vi "Test DI and DO with Troubleshooter.vi"() -> ()   [LabVIEW 2013]
uses:
  SLL DAQ Engine/Software/Source Code/Sub VIs/DAQ Engine/Controls/SLL DE DI Global Options.ctl
  SLL DAQ Engine/Software/Source Code/Sub VIs/DAQ Engine/Controls/SLL DE DO Global Options.ctl
  Controls/ALTS-2015 LV2GBL Station Info Options.ctl
  SLL DAQ Engine/Software/Source Code/Sub VIs/DAQ Engine/Controls/SLL DE List of Digital Inputs.ctl
  SLL DAQ Engine/Software/Source Code/Sub VIs/DAQ Engine/Controls/SLL DE List of Digital Outputs.ctl
  Controls/ALTS-2015 Auto Program States.ctl
panel:
  out "St4 Select Test":bool
  out "St3 Select Test":bool
  out "St2 Select Test":bool
  out "St1 Select Test":bool
  out "St4 Status":bool caption="Status"
  out "St4 Start/Stop":bool
  in  "STATION4 TC FAIL":bool
  in  "STATION4 TC PASS":bool
  out "St4 Test Result":bool caption="Test Result"
  in  "STATION4 Test Type":T1(ring)
  in  "STATION4 Clamped":bool
  in  "STATION4 Stop":bool
  in  "STATION4 Start":bool
  out "St2 Status":bool caption="Status"
  out "St2 Start/Stop":bool
  in  "STATION2 TC FAIL":bool
  in  "STATION2 TC PASS":bool
  out "St2 Test Result":bool caption="Test Result"
  in  "STATION2 Test Type":T1(ring)
  in  "STATION2 Clamped":bool
  in  "STATION2 Stop":bool
  in  "STATION2 Start":bool
  out "St3 Status":bool caption="Status"
  out "St3 Start/Stop":bool
  in  "STATION3 TC FAIL":bool
  in  "STATION3 TC PASS":bool
  out "St3 Test Result":bool caption="Test Result"
  in  "STATION3 Test Type":T1(ring)
  in  "STATION3 Clamped":bool
  in  "STATION3 Stop":bool
  in  "STATION3 Start":bool
  in  "Enum":T2=enum."Write Task Available for Robot"
  in  "Trigger Robot Controller State":bool
  out "St1 Status":bool caption="Status"
  in  "PC ACK Read Tags":dbl
  out "Invalid Serial Number":bool
  out "Rerun?":bool
  out "Station Number":string
  out "Test Result":bool
  out "Serial Flange Size":string
  out "Serial Displacement Size":dbl
  out "Serial Adapter Plate Size":dbl
  out "New Serial Task?":bool
  out "Task Available for Robot?":bool
  in  "Robot Available":bool
  in  "Station No Start Stop Test":T3(ring)
  in  "Scan Trigger":bool
  in  "Stop Test":bool
  in  "Start Test":bool
  out "St1 Start/Stop":bool
  in  "STATION1 TC FAIL":bool
  in  "STATION1 TC PASS":bool
  out "St1 Test Result":bool caption="Test Result"
  in  "STATION1 Test Type":T1(ring)
  in  "STATION1 Clamped":bool
  in  "STATION1 Stop":bool
  in  "STATION1 Start":bool
  out "Station Number":string
  in  "PC_ACK_Read_Tags":dbl
  out "Test Type":i32
  out "DO Channel Name":T4
  out "String":string
  in  "Invalid_SNo":dbl
  in  "Station_No_Start_Stop_Test":dbl
  in  "Start_Test":dbl
  in  "Rerun":dbl
  in  "Station_Number":dbl
  in  "Test_Result":dbl
  in  "Serial_Flange_Size":string
  in  "Serial_Displacement_Size":dbl
  in  "Serial_Adapter_Size":dbl
  in  "New_Serial":dbl
  in  "Scan_Trigger":dbl
  in  "Stop_Test":dbl
  in  "Task_Available_for_Robot":dbl
  in  "Robot_Available":dbl
  in  "DI Array":bool[](array[boolean])=[FALSE, FALSE, FALSE, FALSE, FALSE, FALSE, FALSE, FALSE, FALSE, FALSE, FALSE, FALSE, FALSE, FALSE, FALSE, FALSE, FALSE, FALSE, FALSE, FALSE, FALSE, FALSE, FALSE, FALSE, FALSE, FALSE, FALSE, FALSE]
  in  "DI Channel Name Array":T5[](array[typedef])=[enum."STATION1_START", enum."STATION1_STOP", enum."STATION1_CLAMPED", enum."STATION1_TC_PASS", enum."STATION1_TC_FAIL", enum."STATION1_TTA", enum."STATION1_TTB", enum."STATION2_START", enum."STATION2_STOP", enum."STATION2_CLAMPED", enum."STATION2_TC_PASS", enum."STATION2_TC_FAIL", enum."STATION2_TTA", enum."STATION2_TTB", enum."STATION3_START", enum."STATION3_STOP", enum."STATION3_CLAMPED", enum."STATION3_TC_PASS", enum."STATION3_TC_FAIL", enum."STATION3_TTA", enum."STATION3_TTB", enum."STATION4_START", enum."STATION4_STOP", enum."STATION4_CLAMPED", enum."STATION4_TC_PASS", enum."STATION4_TC_FAIL", enum."STATION4_TTA", enum."STATION4_TTB"]
  out "DO Channel Name Array":T4[](array[typedef])=[enum."STATION1_START TEST", enum."STATION1_STOP TEST", enum."STATION1_LIGHT1", enum."STATION1_LIGHT2", enum."STATION1_LIGHT3", enum."STATION1_SELECT_TEST", enum."STATION2_START TEST", enum."STATION2_STOP TEST", enum."STATION2_LIGHT1", enum."STATION2_LIGHT2", enum."STATION2_LIGHT3", enum."STATION2_SELECT_TEST", enum."STATION3_START TEST", enum."STATION3_STOP TEST", enum."STATION3_LIGHT1", enum."STATION3_LIGHT2", enum."STATION3_LIGHT3", enum."STATION3_SELECT_TEST", enum."STATION4_START TEST", enum."STATION4_STOP TEST", enum."STATION4_LIGHT1", enum."STATION4_LIGHT2", enum."STATION4_LIGHT3", enum."STATION4_SELECT_TEST"]
  out "DO Status":bool[](array[boolean])
  out "error out":errorcluster
  in  "error in":errorcluster
  in  "DI Channel Name":T5
  in  "stop":bool
  # "STATION  1"
  # "STATION  2"
  # "Write Tags\nPC Writes to PLC\nPLC can only read these tags"
  # "Read Tags\nPC Reads from PLC"
  # "DO"
  # "DO"
  # "DO"
  # "DO"
  # "STATION  3"
  # "STATION  4"
  # "DO"
  # "DO"
  # "DO"
  # "DO"
  # "TROUBLESHOOTER"
  # "Simulation VI to send DI Status and reads the DO output"
  # "Write Tags\nPC Writes to PLC\nPLC can only read these tags"
  # "Read Tags\nPC Reads from PLC"
  # "Test Type1: TTA:1, TTB: 0;\nTest Type2: TTA:0, TTB: 1;\nTest Type3: TTA:1, TTB: 1;\nTest Type4: TTA:0, TTB: 0;"
  # "IDLE : \t\t100\nTest Running:\t 010\nPass\t\t110\nFail\t\t101"
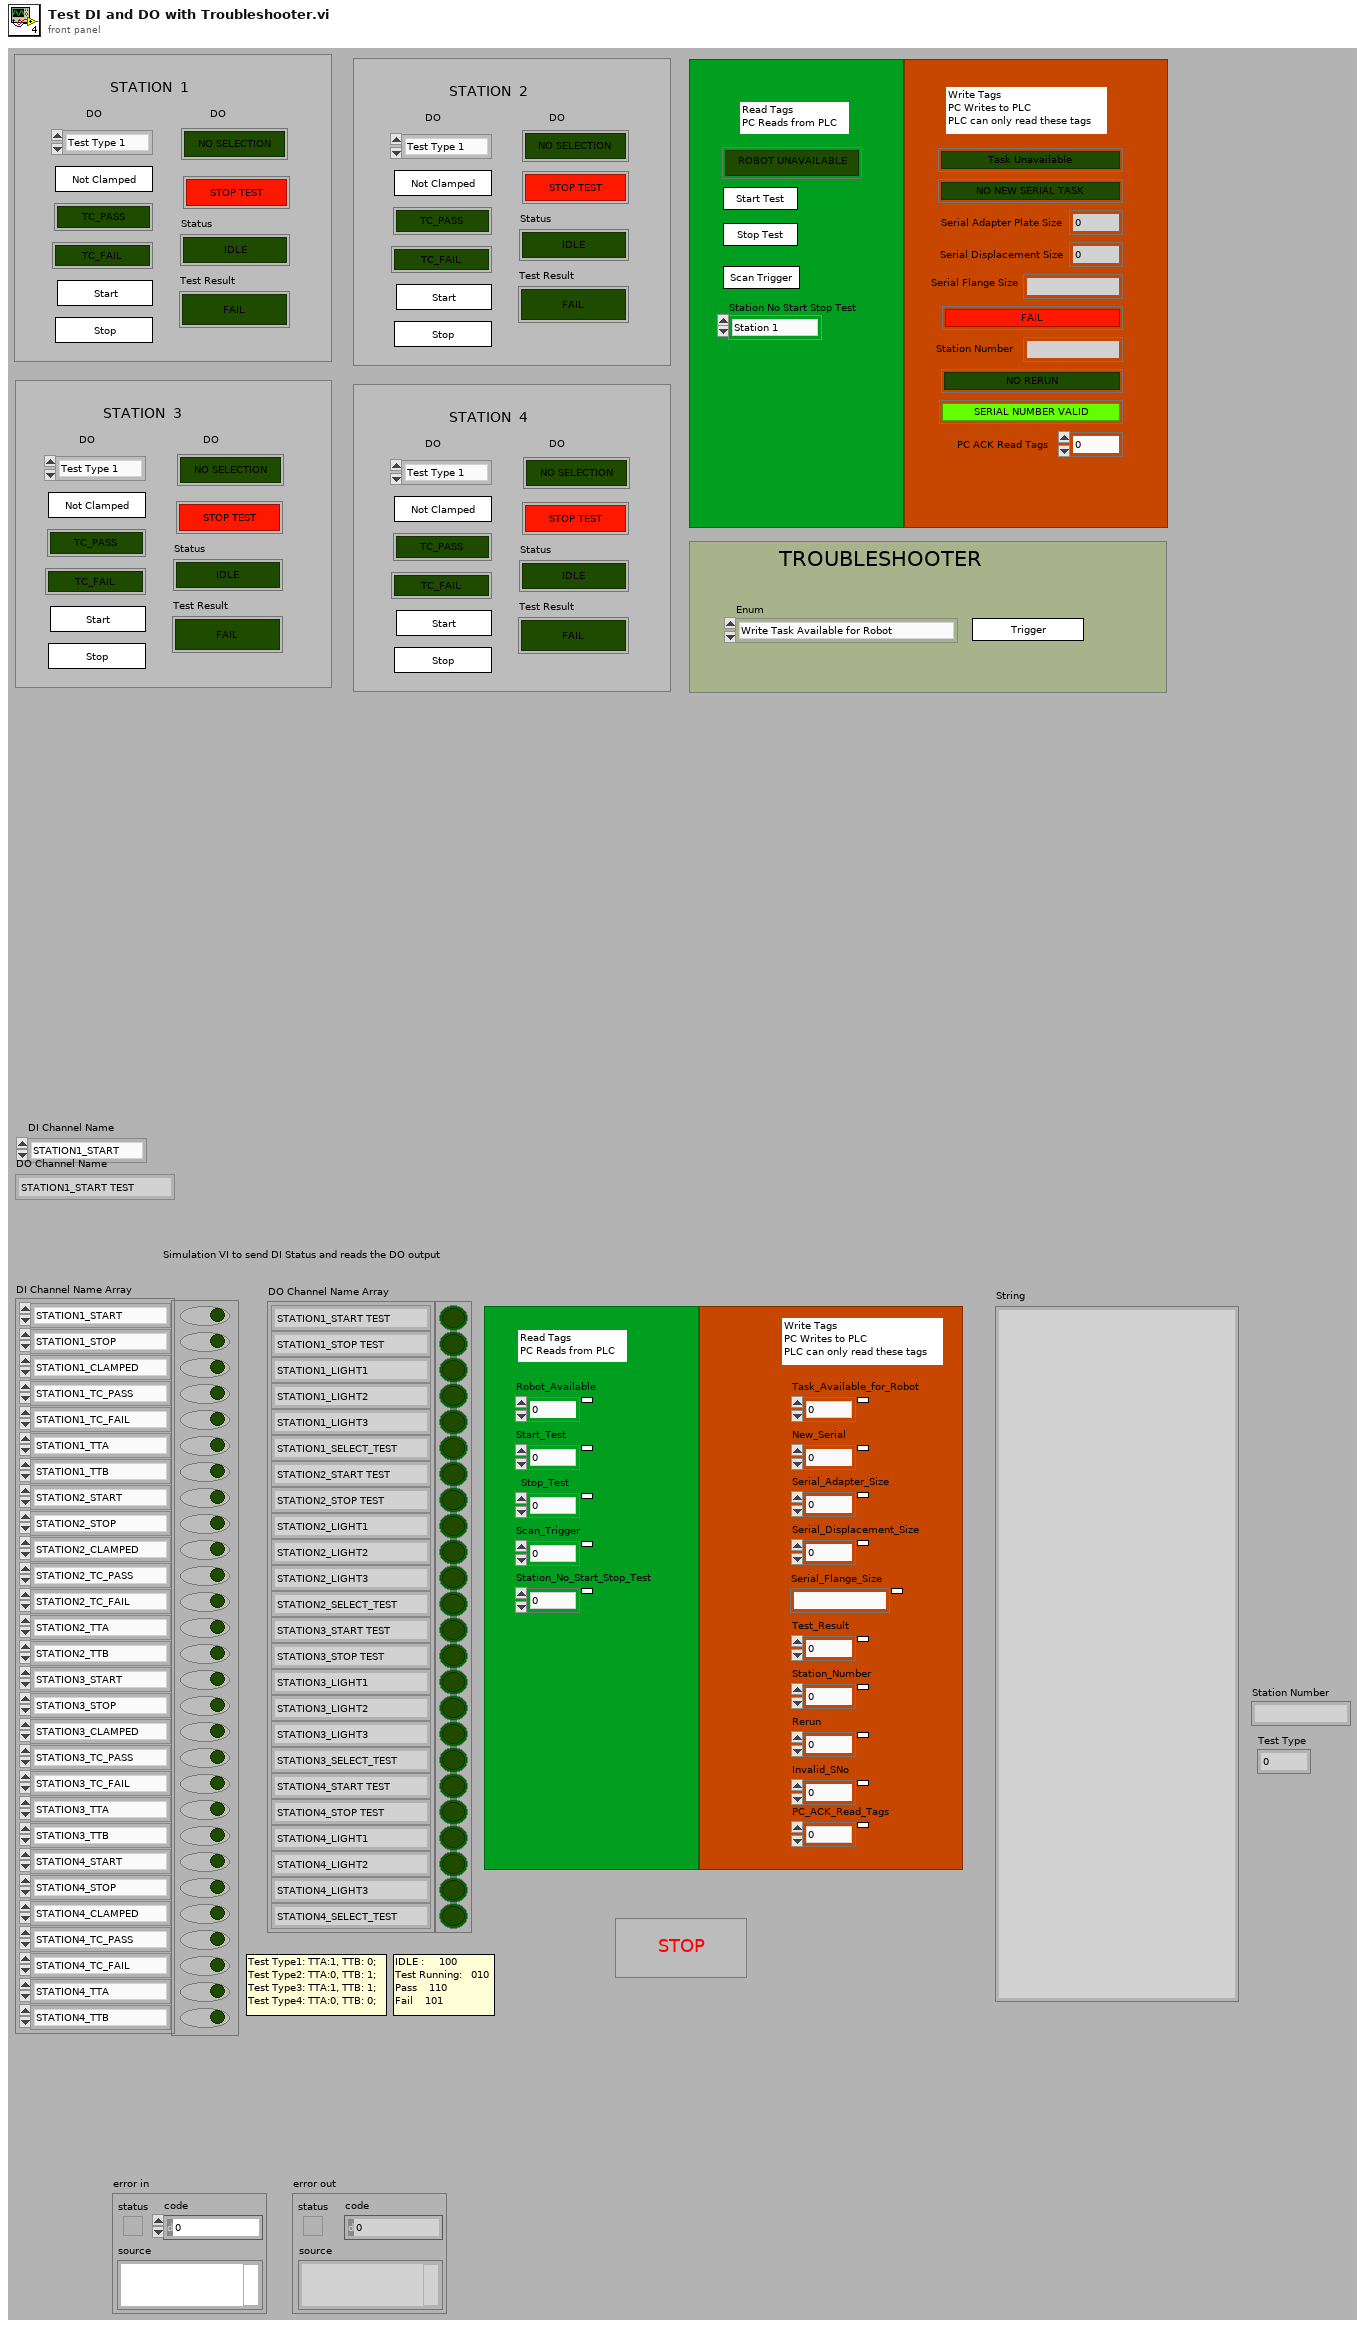
[diagram p1: front panel]
types:
  T1 = enum16{"Test Type 1", "Test Type 2", "Test Type 3", "Test Type 4"}
  T2 = typedef "ALTS-2015 Auto Program States.ctl" = enum16{"<------ Robot Handler States ------>", "Wait for Robot Availability", "Wait & Read Task from Queue", "Write New Task Details to Robot", "Write Task Available for Robot", "Check Robot for Unavailbilty", "Write Task Unavailable for Robot", "<------------ Other ------------>", "Error", "Exit"}
  T3 = enum16{"Station 1", "Station 2", "Station 3", "Station 4"}
  T4 = typedef "SLL DE List of Digital Outputs.ctl" = enum16{"STATION1_START TEST", "STATION1_STOP TEST", "STATION1_LIGHT1", "STATION1_LIGHT2", "STATION1_LIGHT3", "STATION1_SELECT_TEST", "STATION2_START TEST", "STATION2_STOP TEST", "STATION2_LIGHT1", "STATION2_LIGHT2", "STATION2_LIGHT3", "STATION2_SELECT_TEST", "STATION3_START TEST", "STATION3_STOP TEST", "STATION3_LIGHT1", "STATION3_LIGHT2", "STATION3_LIGHT3", "STATION3_SELECT_TEST", "STATION4_START TEST", "STATION4_STOP TEST", "STATION4_LIGHT1", "STATION4_LIGHT2", "STATION4_LIGHT3", "STATION4_SELECT_TEST"}
  T5 = typedef "SLL DE List of Digital Inputs.ctl" = enum16{"STATION1_START", "STATION1_STOP", "STATION1_CLAMPED", "STATION1_TC_PASS", "STATION1_TC_FAIL", "STATION1_TTA", "STATION1_TTB", "STATION2_START", "STATION2_STOP", "STATION2_CLAMPED", "STATION2_TC_PASS", "STATION2_TC_FAIL", "STATION2_TTA", "STATION2_TTB", "STATION3_START", "STATION3_STOP", "STATION3_CLAMPED", "STATION3_TC_PASS", "STATION3_TC_FAIL", "STATION3_TTA", "STATION3_TTB", "STATION4_START", "STATION4_STOP", "STATION4_CLAMPED", "STATION4_TC_PASS", "STATION4_TC_FAIL", "STATION4_TTA", "STATION4_TTB"}
  T6 = enum32{"No PSP", "Read", "Write", "Write & Read"}
  T7 = typedef "ALTS-2015 LV2GBL Station Info Options.ctl" = enum16{"Init", "Read", "Read All", "Write Sensor ID", "Write  Work Order", "Write Serial Number", "Write Test Data", "Write Station Status", "Write Station Occupancy", "Write Station Test Type", "Write Rerun", "Clear All", "Clear Test Result"}
  T8 = typedef "SLL DE DO Global Options.ctl" = enum16{"Init", "Write Line", "Write Array", "Write Full Status", "Read Line", "Read Array", "Read Full Status", "Restart DO", "Send to Safe Mode", "Stop DO"}
  T9 = typedef "SLL DE DI Global Options.ctl" = enum16{"Init", "Write Line", "Write Array", "Read Line", "Read Array", "Read Full Status", "Write Full Status"}
  T10 = typedef "ALTS-2015 Station Details.ctl" = cluster{"Station Number":string, "Work Order Number":string, "Sensor Name":string, "Pressure (PSI)":string, "Flow (SCCM)":string, "Test Time ":string, "Test Result":string, "Serial Number":string, "Station Status":T11, "Station Occupied?":bool, "Rerun Count":i32, "Test Type":i32}
  T11 = typedef "ALTS-2015 Status Ring Indicator.ctl" = u16
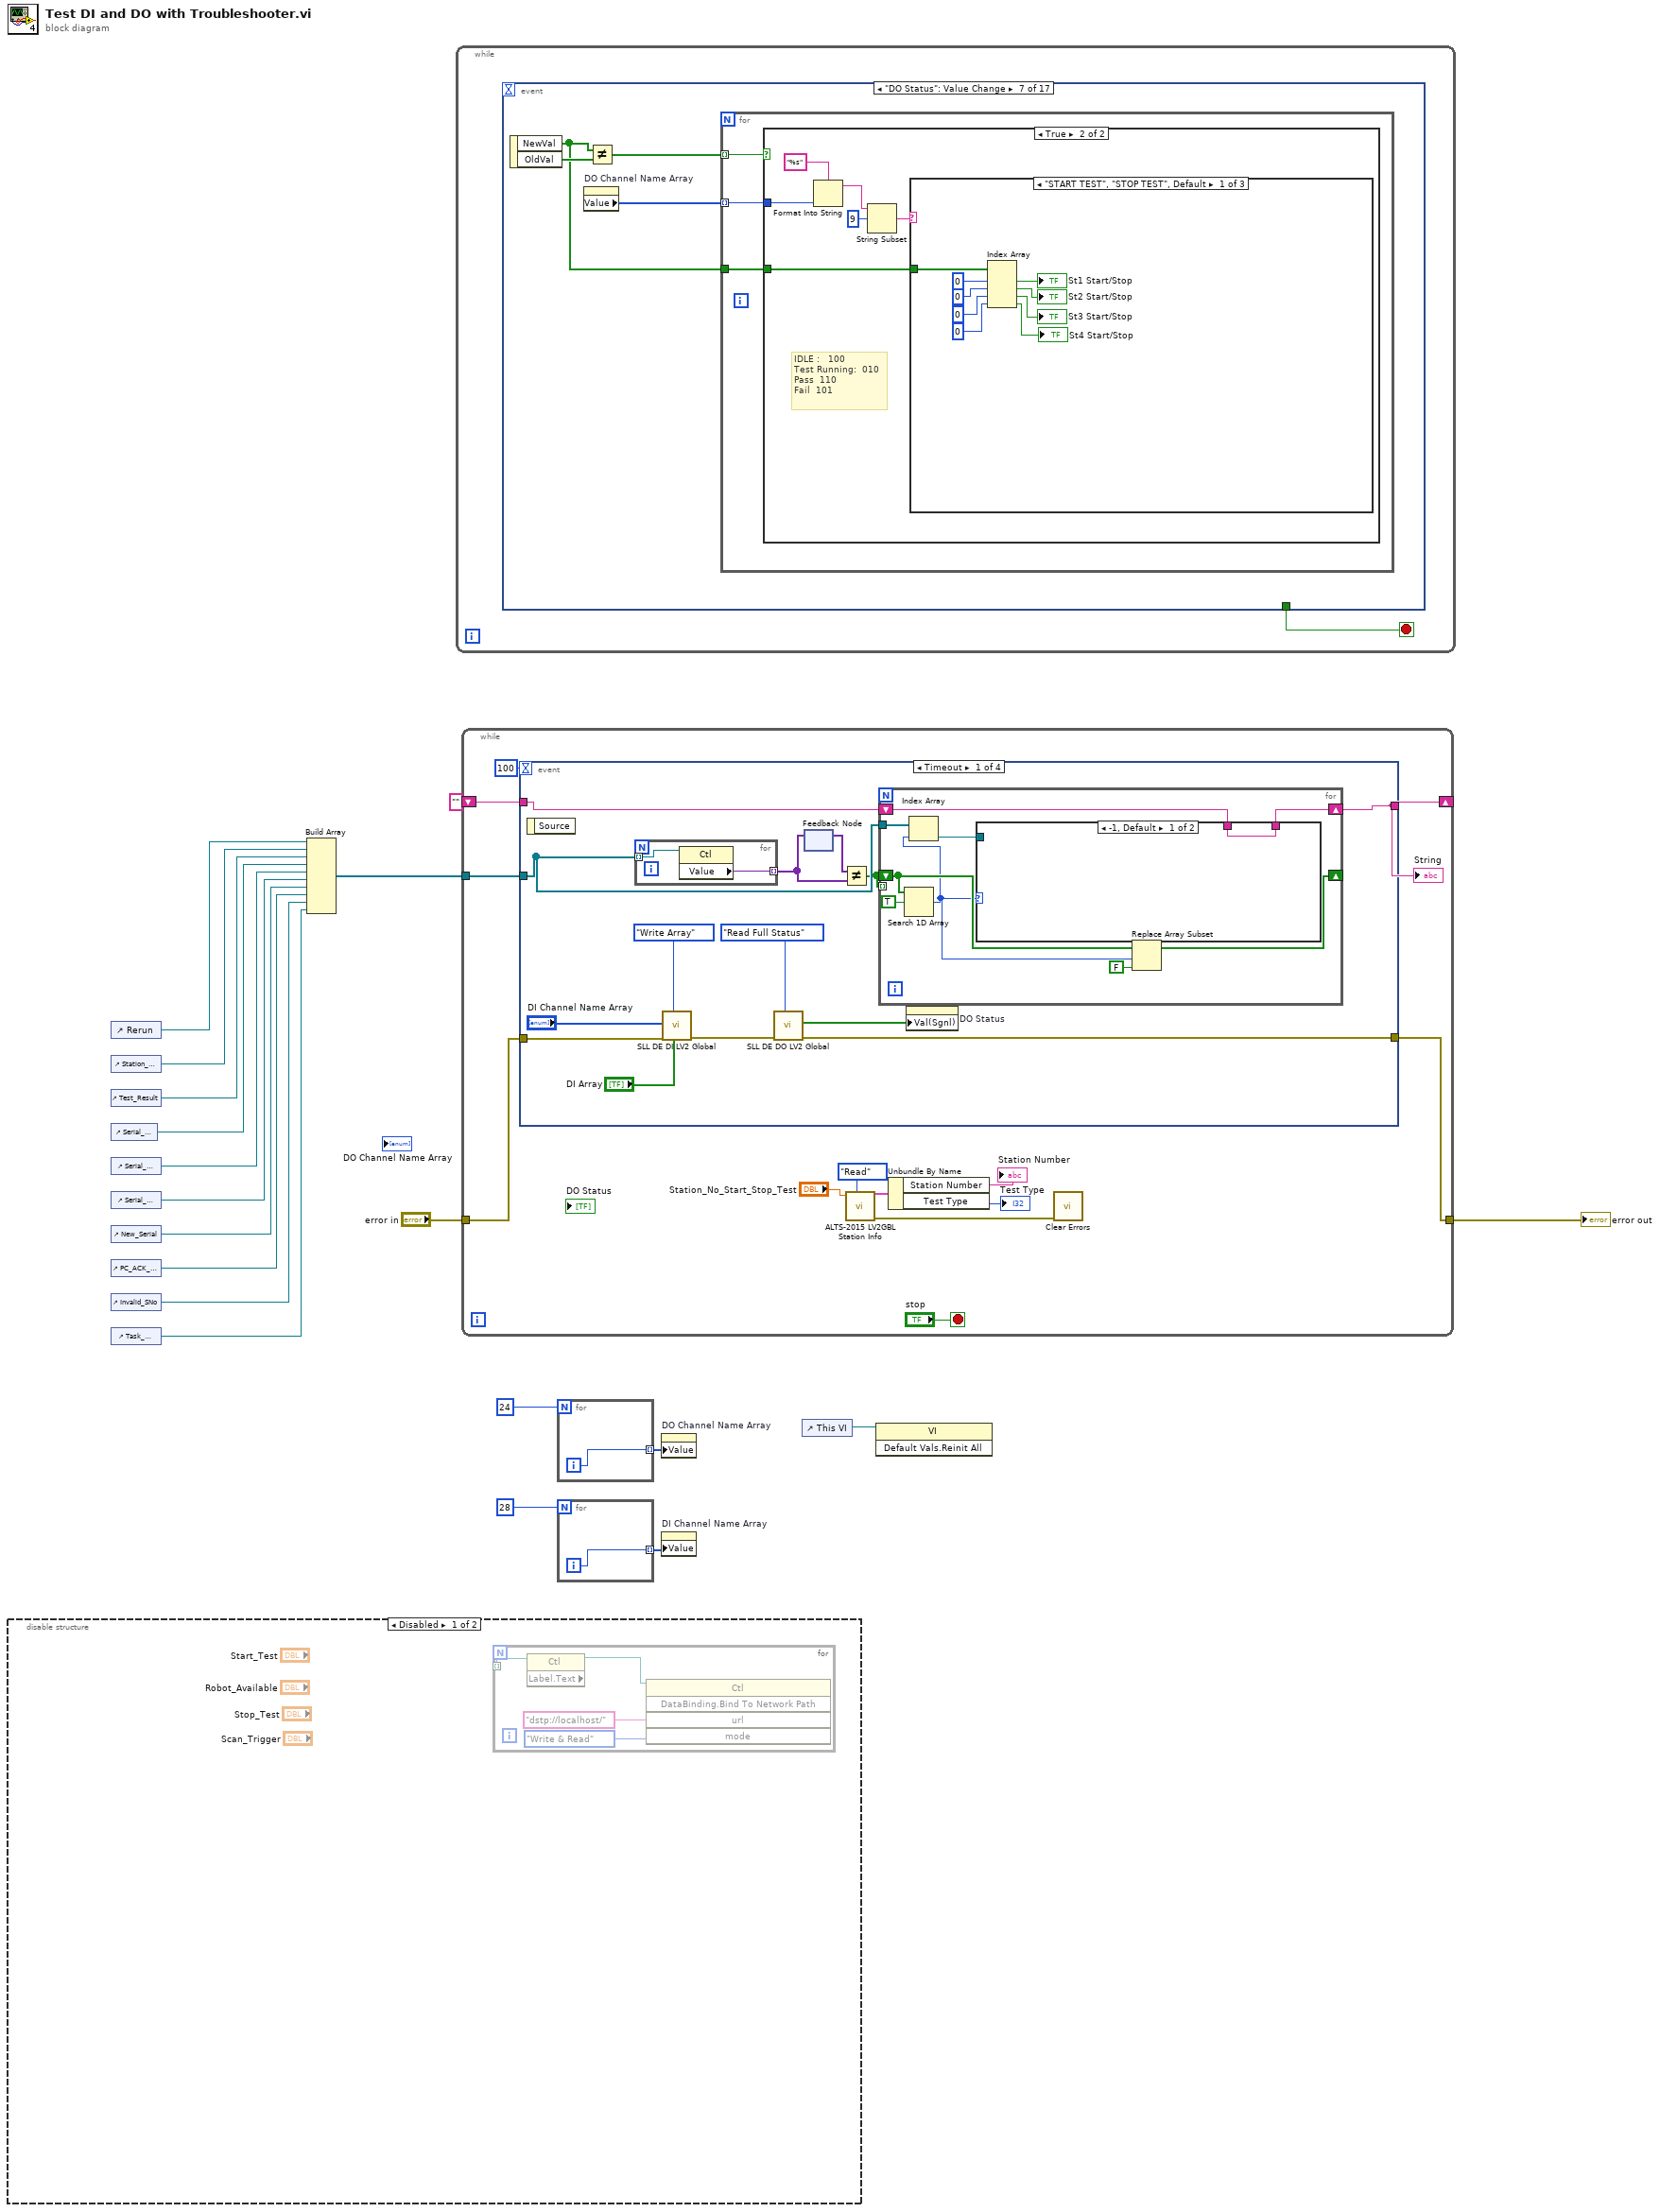
[diagram p0: block diagram]
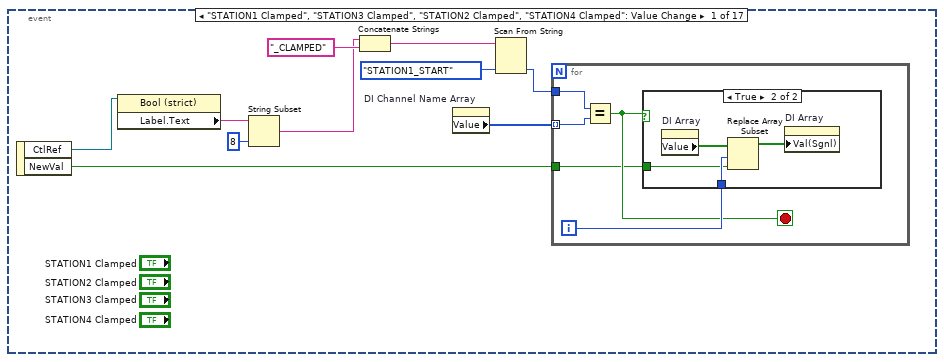
[diagram p2: hidden frame]
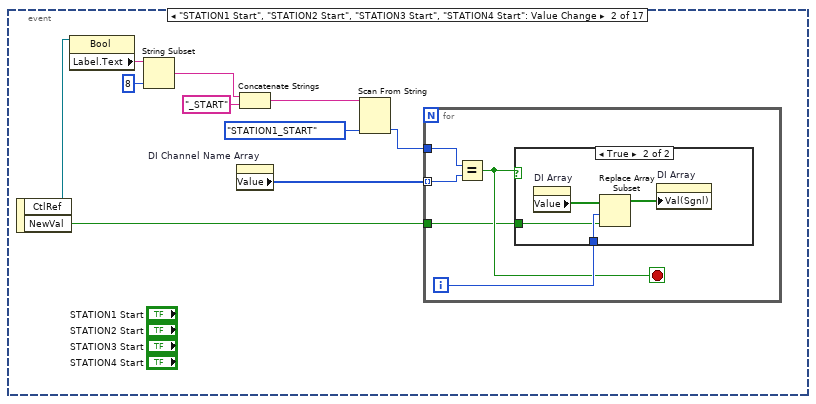
[diagram p4: hidden frame]
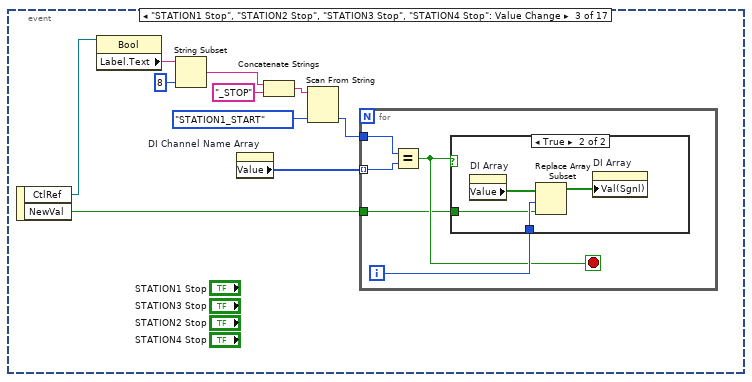
[diagram p6: hidden frame]
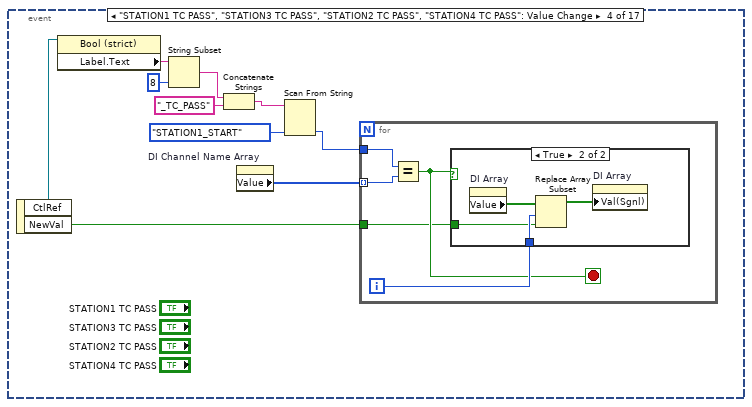
[diagram p8: hidden frame]
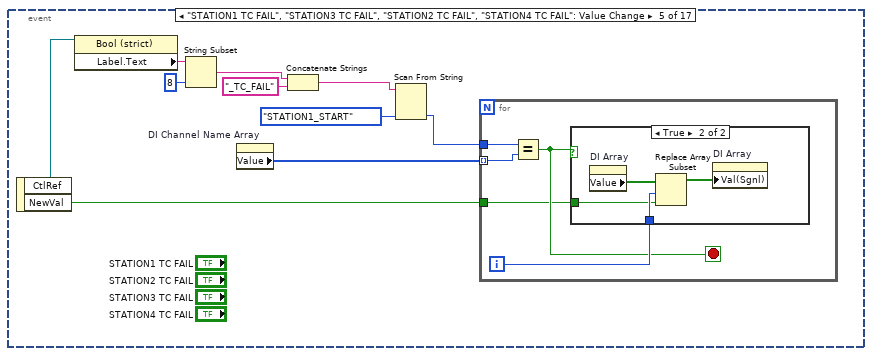
[diagram p10: hidden frame]
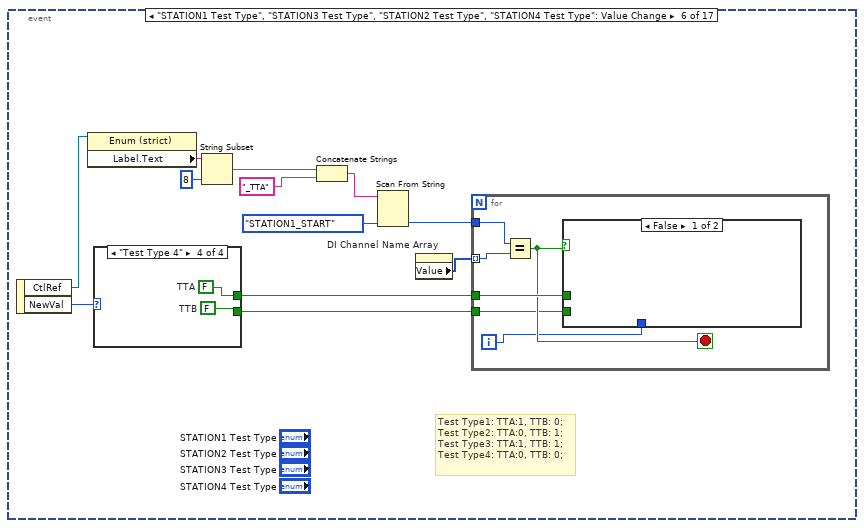
[diagram p12: hidden frame]
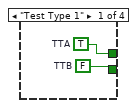
[diagram p13: hidden frame]
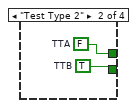
[diagram p14: hidden frame]
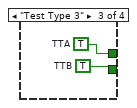
[diagram p15: hidden frame]
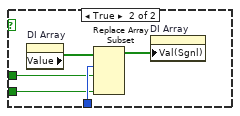
[diagram p16: hidden frame]
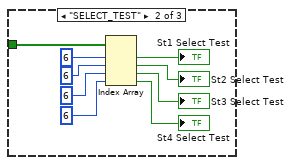
[diagram p18: hidden frame]
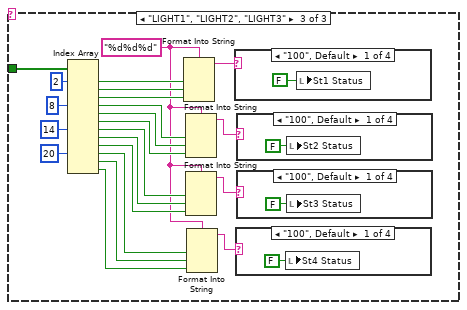
[diagram p19: hidden frame]
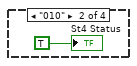
[diagram p20: hidden frame]
diagram:
  n1 = disable-structure shown="Disabled" {
    frame Disabled {
      n2 = for {
        tunnel: [w24] -> w20 mode=indexing
        n3 = property class="Ctl" props=["Label", "Text"](reference=w24) -> (reference out=w21:refnum<vi>)  [unwired: 1 in, 2 out]
        n4 = invoke on="Invoke Node" class="Ctl" method="DataBinding.Bind To Network Path"(reference=w21, "url"="dstp://localhost/" ("URL"), "mode"=T6."Write & Read" ("Mode")) -> ()  [unwired: 2 in, 5 out]
      }
    }
    frame Enabled {
    }
  }
  n5 = control-ref of="Rerun"() -> (w3:refnum<vi>)
  n6 = control-ref of="Station_Number"() -> (w4:refnum<vi>)
  n7 = control-ref of="Test_Result"() -> (w5:refnum<vi>)
  n8 = control-ref of="Serial_Flange_Size"() -> (w6:refnum<vi>)
  n9 = control-ref of="Serial_Displacement_Size"() -> (w7:refnum<vi>)
  n10 = control-ref of="Serial_Adapter_Size"() -> (w8:refnum<vi>)
  n11 = control-ref of="New_Serial"() -> (w9:refnum<vi>)
  n12 = control-ref of="PC_ACK_Read_Tags"() -> (w1:refnum<vi>)
  n13 = control-ref of="Invalid_SNo"() -> (w10:refnum<vi>)
  n14 = control-ref of="Task_Available_for_Robot"() -> (w11:refnum<vi>)
  n15 = Build Array(w3, w4, w5, w6, w7, w8, w9, w1, w10, w11) -> (w2:refnum<vi>[])
  n16 = while {
    stop <- w25 stop-if-true
    n17 = event shown="[6] \"DO Status\": Value Change" {
      selector: _ -> [_ _ _ _ _ _ _ _ _ _ _ _ _ _ _ _ _]
      dyn-events: _ -> [_ _ _ _ _ _ _ _ _ _ _ _ _ _ _ _ _]
      timeout: _ -> [_ _ _ _ _ _ _ _ _ _ _ _ _ _ _ _ _]
      tunnel: [_ _ _ _ _ _ _ _ _ _ _ _ _ _ _ TRUE _] -> w25
      event "STATION1 Clamped", "STATION3 Clamped", "STATION2 Clamped", "STATION4 Clamped": Value Change {
        n18 = event-data() -> ("CtlRef"=w32:refnum<vi>, "NewVal"=w33:bool)  [unwired: 1 in]
        n19 = property class="Bool (strict)"(reference=w32) -> ("Label.Text"=w31:string)  [unwired: 1 in, 2 out]
        n20 = String Subset(string=w31, length (rest)=8 ("length (rest)")) -> (substring=w30:string)  [unwired: 1 in]
        n21 = Concatenate Strings(w30, "_CLAMPED" ("string")) -> (w28:string)
        n22 = property on="DI Channel Name Array" class="Arr (strict)"() -> ("Value"=w34:T5[])  [unwired: 2 in, 2 out]
        n23 = Scan From String(input string=w28, default 1=SLL_DE_List_of_Digital_Inputs."STATION1_START" ("List of Digital Inputs")) -> (output 1=w27:T5)  [unwired: 3 in, 3 out]
        n24 = for {
          tunnel: w27 -> [w40]
          tunnel: w34 -> [w39] mode=indexing
          tunnel: w33 -> [w36]
          i -> [w38]
          stop <- w37 stop-if-true
          n25 = Equal?(x=w40, y=w39) -> (x = y?=w37:bool)
          n26 = case shown="True" w37 {
            tunnel: w38 -> [_ w43]
            tunnel: w36 -> [_ w41]
            frame False {
            }
            frame True {
              n27 = property on="DI Array" class="Arr (strict)"() -> ("Value"=w44:bool[])  [unwired: 2 in, 2 out]
              n28 = Replace Array Subset(array=w44, new element=w41, index=w43) -> (w42:bool[])
              n29 = property on="DI Array" class="Arr (strict)"("Val(Sgnl)"=w42) -> ()  [unwired: 2 in, 2 out]
            }
          }
        }
      }
      event "STATION1 Start", "STATION2 Start", "STATION3 Start", "STATION4 Start": Value Change {
        n30 = event-data() -> ("CtlRef"=w51:refnum<vi>, "NewVal"=w52:bool)  [unwired: 1 in]
        n31 = property class="Bool"(reference=w51) -> ("Label.Text"=w50:string)  [unwired: 1 in, 2 out]
        n32 = String Subset(string=w50, length (rest)=8 ("length (rest)")) -> (substring=w48:string)  [unwired: 1 in]
        n33 = property on="DI Channel Name Array" class="Arr (strict)"() -> ("Value"=w53:T5[])  [unwired: 2 in, 2 out]
        n34 = Concatenate Strings(w48, "_START" ("string")) -> (w47:string)
        n35 = Scan From String(input string=w47, default 1=SLL_DE_List_of_Digital_Inputs."STATION1_START" ("List of Digital Inputs")) -> (output 1=w45:T5)  [unwired: 3 in, 3 out]
        n36 = for {
          tunnel: w45 -> [w59]
          tunnel: w53 -> [w58] mode=indexing
          tunnel: w52 -> [w55]
          i -> [w57]
          stop <- w56 stop-if-true
          n37 = Equal?(x=w59, y=w58) -> (x = y?=w56:bool)
          n38 = case shown="True" w56 {
            tunnel: w57 -> [_ w62]
            tunnel: w55 -> [_ w60]
            frame False {
            }
            frame True {
              n39 = property on="DI Array" class="Arr (strict)"() -> ("Value"=w63:bool[])  [unwired: 2 in, 2 out]
              n40 = Replace Array Subset(array=w63, new element=w60, index=w62) -> (w61:bool[])
              n41 = property on="DI Array" class="Arr (strict)"("Val(Sgnl)"=w61) -> ()  [unwired: 2 in, 2 out]
            }
          }
        }
      }
      event "STATION1 Stop", "STATION2 Stop", "STATION3 Stop", "STATION4 Stop": Value Change {
        n42 = event-data() -> ("CtlRef"=w70:refnum<vi>, "NewVal"=w71:bool)  [unwired: 1 in]
        n43 = property class="Bool"(reference=w70) -> ("Label.Text"=w69:string)  [unwired: 1 in, 2 out]
        n44 = String Subset(string=w69, length (rest)=8 ("length (rest)")) -> (substring=w68:string)  [unwired: 1 in]
        n45 = property on="DI Channel Name Array" class="Arr (strict)"() -> ("Value"=w72:T5[])  [unwired: 2 in, 2 out]
        n46 = Concatenate Strings(w68, "_STOP" ("string")) -> (w66:string)
        n47 = Scan From String(input string=w66, default 1=SLL_DE_List_of_Digital_Inputs."STATION1_START" ("List of Digital Inputs")) -> (output 1=w65:T5)  [unwired: 3 in, 3 out]
        n48 = for {
          tunnel: w65 -> [w78]
          tunnel: w72 -> [w77] mode=indexing
          tunnel: w71 -> [w74]
          i -> [w76]
          stop <- w75 stop-if-true
          n49 = Equal?(x=w78, y=w77) -> (x = y?=w75:bool)
          n50 = case shown="True" w75 {
            tunnel: w76 -> [_ w81]
            tunnel: w74 -> [_ w79]
            frame False {
            }
            frame True {
              n51 = property on="DI Array" class="Arr (strict)"() -> ("Value"=w82:bool[])  [unwired: 2 in, 2 out]
              n52 = Replace Array Subset(array=w82, new element=w79, index=w81) -> (w80:bool[])
              n53 = property on="DI Array" class="Arr (strict)"("Val(Sgnl)"=w80) -> ()  [unwired: 2 in, 2 out]
            }
          }
        }
      }
      event "STATION1 TC PASS", "STATION3 TC PASS", "STATION2 TC PASS", "STATION4 TC PASS": Value Change {
        n54 = event-data() -> ("CtlRef"=w86:refnum<vi>, "NewVal"=w90:bool)  [unwired: 1 in]
        n55 = property class="Bool (strict)"(reference=w86) -> ("Label.Text"=w88:string)  [unwired: 1 in, 2 out]
        n56 = String Subset(string=w88, length (rest)=8 ("length (rest)")) -> (substring=w87:string)  [unwired: 1 in]
        n57 = Concatenate Strings(w87, "_TC_PASS" ("string")) -> (w85:string)
        n58 = property on="DI Channel Name Array" class="Arr (strict)"() -> ("Value"=w91:T5[])  [unwired: 2 in, 2 out]
        n59 = Scan From String(input string=w85, default 1=SLL_DE_List_of_Digital_Inputs."STATION1_START" ("List of Digital Inputs")) -> (output 1=w83:T5)  [unwired: 3 in, 3 out]
        n60 = for {
          tunnel: w83 -> [w97]
          tunnel: w91 -> [w96] mode=indexing
          tunnel: w90 -> [w93]
          i -> [w95]
          stop <- w94 stop-if-true
          n61 = Equal?(x=w97, y=w96) -> (x = y?=w94:bool)
          n62 = case shown="True" w94 {
            tunnel: w95 -> [_ w100]
            tunnel: w93 -> [_ w98]
            frame False {
            }
            frame True {
              n63 = property on="DI Array" class="Arr (strict)"() -> ("Value"=w101:bool[])  [unwired: 2 in, 2 out]
              n64 = Replace Array Subset(array=w101, new element=w98, index=w100) -> (w99:bool[])
              n65 = property on="DI Array" class="Arr (strict)"("Val(Sgnl)"=w99) -> ()  [unwired: 2 in, 2 out]
            }
          }
        }
      }
      event "STATION1 TC FAIL", "STATION3 TC FAIL", "STATION2 TC FAIL", "STATION4 TC FAIL": Value Change {
        n66 = event-data() -> ("CtlRef"=w106:refnum<vi>, "NewVal"=w109:bool)  [unwired: 1 in]
        n67 = property class="Bool (strict)"(reference=w106) -> ("Label.Text"=w107:string)  [unwired: 1 in, 2 out]
        n68 = String Subset(string=w107, length (rest)=8 ("length (rest)")) -> (substring=w105:string)  [unwired: 1 in]
        n69 = property on="DI Channel Name Array" class="Arr (strict)"() -> ("Value"=w110:T5[])  [unwired: 2 in, 2 out]
        n70 = Concatenate Strings(w105, "_TC_FAIL" ("string")) -> (w104:string)
        n71 = Scan From String(input string=w104, default 1=SLL_DE_List_of_Digital_Inputs."STATION1_START" ("List of Digital Inputs")) -> (output 1=w102:T5)  [unwired: 3 in, 3 out]
        n72 = for {
          tunnel: w110 -> [w116] mode=indexing
          tunnel: w109 -> [w113]
          tunnel: w102 -> [w112]
          i -> [w115]
          stop <- w114 stop-if-true
          n73 = Equal?(x=w112, y=w116) -> (x = y?=w114:bool)
          n74 = case shown="True" w114 {
            tunnel: w115 -> [_ w119]
            tunnel: w113 -> [_ w117]
            frame False {
            }
            frame True {
              n75 = property on="DI Array" class="Arr (strict)"() -> ("Value"=w120:bool[])  [unwired: 2 in, 2 out]
              n76 = Replace Array Subset(array=w120, new element=w117, index=w119) -> (w118:bool[])
              n77 = property on="DI Array" class="Arr (strict)"("Val(Sgnl)"=w118) -> ()  [unwired: 2 in, 2 out]
            }
          }
        }
      }
      event "STATION1 Test Type", "STATION3 Test Type", "STATION2 Test Type", "STATION4 Test Type": Value Change {
        # "Test Type1: TTA:1, TTB: 0;\nTest Type2: TTA:0, TTB: 1;\nTest Type3: TTA:1, TTB: 1;\nTest Type4: TTA:0, TTB: 0;"
        n78 = event-data() -> ("CtlRef"=w125:refnum<vi>, "NewVal"=w130:T1)  [unwired: 1 in]
        n79 = property class="Enum (strict)"(reference=w125) -> ("Label.Text"=w127:string)  [unwired: 1 in, 2 out]
        n80 = case shown="\"Test Type 4\"" w130 {
          tunnel: [w134 w136 w138 w140] -> w129
          tunnel: [w133 w135 w137 w139] -> w128
          frame "Test Type 1" {
            w133 = FALSE  # TTB
            w134 = TRUE  # TTA
          }
          frame "Test Type 2" {
            w135 = TRUE  # TTB
            w136 = FALSE  # TTA
          }
          frame "Test Type 3" {
            w137 = TRUE  # TTB
            w138 = TRUE  # TTA
          }
          frame "Test Type 4" {
            w139 = FALSE  # TTB
            w140 = FALSE  # TTA
          }
        }
        n81 = String Subset(string=w127, length (rest)=8 ("length (rest)")) -> (substring=w126:string)  [unwired: 1 in]
        n82 = Concatenate Strings(w126, "_TTA" ("string")) -> (w123:string)
        n83 = Scan From String(input string=w123, default 1=SLL_DE_List_of_Digital_Inputs."STATION1_START" ("List of Digital Inputs")) -> (output 1=w122:T5)  [unwired: 3 in, 3 out]
        n84 = property on="DI Channel Name Array" class="Arr (strict)"() -> ("Value"=w131:T5[])  [unwired: 2 in, 2 out]
        n85 = for {
          tunnel: w122 -> [w146]
          tunnel: w131 -> [w145] mode=indexing
          tunnel: w129 -> [w144]
          tunnel: w128 -> [w141]
          i -> [w142]
          stop <- w143 stop-if-true
          n86 = Equal?(x=w146, y=w145) -> (x = y?=w143:bool)
          n87 = case shown="False" w143 {
            tunnel: w142 -> [_ w150]
            tunnel: w144 -> [_ w148]
            tunnel: w141 -> [_ w147]
            frame False {
            }
            frame True {
              n88 = property on="DI Array" class="Arr (strict)"() -> ("Value"=w151:bool[])  [unwired: 2 in, 2 out]
              n89 = Replace Array Subset(array=w151, new element #1=w148, index #1=w150, new element #2=w147) -> (w149:bool[])  [unwired: 1 in]
              n90 = property on="DI Array" class="Arr (strict)"("Val(Sgnl)"=w149) -> ()  [unwired: 2 in, 2 out]
            }
          }
        }
      }
      event "DO Status": Value Change {
        n91 = event-data() -> ("NewVal"=w152:bool[], "OldVal"=w155:bool[])  [unwired: 1 in]
        n92 = property on="DO Channel Name Array" class="Arr (strict)"() -> ("Value"=w153:T4[])  [unwired: 2 in, 2 out]
        n93 = Not Equal?(x=w152, y=w155) -> (x != y?=w154:bool[])
        n94 = for {
          tunnel: w154 -> [w158] mode=indexing
          tunnel: w153 -> [w157] mode=indexing
          tunnel: w152 -> [w156]
          n95 = case shown="True" w158 {
            tunnel: w157 -> [_ w164]
            tunnel: w156 -> [_ w159]
            frame False {
            }
            frame True {
              # "IDLE : \t\t100\nTest Running:\t 010\nPass\t\t110\nFail\t\t101"
              n96 = Format Into String(format string="%s", w164) -> (resulting string=w160:string)  [unwired: 2 in, 1 out]
              n97 = String Subset(string=w160, offset (0)=9 ("length (rest)")) -> (substring=w161:string)  [unwired: 1 in]
              n98 = case shown="\"START TEST\", \"STOP TEST\", Default" w161 {
                tunnel: w159 -> [w173 w182 w204]
                frame "START TEST", "STOP TEST", Default {
                  n99 = Index Array(array=w173, index #1=0 ("index"), index #2=0 ("index"), index #3=0 ("index"), index #4=0 ("index")) -> (element #1=→"St1 Start/Stop":bool, element #2=→"St2 Start/Stop":bool, element #3=→"St3 Start/Stop":bool, element #4=→"St4 Start/Stop":bool)
                }
                frame "SELECT_TEST" {
                  n100 = Index Array(array=w182, index #1=6 ("index"), index #2=6 ("index"), index #3=6 ("index"), index #4=6 ("index")) -> (element #1=→"St1 Select Test":bool, element #2=→"St2 Select Test":bool, element #3=→"St3 Select Test":bool, element #4=→"St4 Select Test":bool)
                }
                frame "LIGHT1", "LIGHT2", "LIGHT3" {
                  w187 = "%d%d%d" ("format string")
                  n101 = Index Array(array=w204, index #1=2 ("index"), index #4=8 ("index"), index #7=14 ("index"), index #10=20 ("index")) -> (element #1=w199:bool, element #2=w198:bool, element #3=w197:bool, element #4=w196:bool, element #5=w195:bool, element #6=w194:bool, element #7=w193:bool, element #8=w192:bool, element #9=w190:bool, element #10=w191:bool, element #11=w189:bool, element #12=w188:bool)  [unwired: 8 in]
                  n102 = Format Into String(format string=w187, w199, w198, w197) -> (resulting string=w186:string)  [unwired: 2 in, 1 out]
                  n103 = Format Into String(format string=w187, w196, w195, w194) -> (resulting string=w185:string)  [unwired: 2 in, 1 out]
                  n104 = Format Into String(format string=w187, w193, w192, w190) -> (resulting string=w183:string)  [unwired: 2 in, 1 out]
                  n105 = Format Into String(format string=w187, w191, w189, w188) -> (resulting string=w184:string)  [unwired: 2 in, 1 out]
                  n106 = case shown="\"100\", Default" w186 {
                    frame "100", Default {
                      n107 = local write "St1 Status"(FALSE ("Running?")) -> ()
                    }
                    frame "010" {
                      "St1 Status" <- TRUE ("Running?")
                    }
                    frame "110" {
                      "St1 Test Result" <- TRUE ("St1 Test Result")
                    }
                    frame "101" {
                      n108 = local write "St1 Test Result"(FALSE ("St1 Test Result")) -> ()
                    }
                  }
                  n109 = case shown="\"100\", Default" w184 {
                    frame "100", Default {
                      n110 = local write "St4 Status"(FALSE ("Running?")) -> ()
                    }
                    frame "010" {
                      "St4 Status" <- TRUE ("Running?")
                    }
                    frame "110" {
                      "St4 Test Result" <- TRUE ("St1 Test Result")
                    }
                    frame "101" {
                      n111 = local write "St4 Test Result"(FALSE ("St1 Test Result")) -> ()
                    }
                  }
                  n112 = case shown="\"100\", Default" w185 {
                    frame "100", Default {
                      n113 = local write "St2 Status"(FALSE ("Running?")) -> ()
                    }
                    frame "010" {
                      "St2 Status" <- TRUE ("Running?")
                    }
                    frame "110" {
                      n114 = local write "St2 Test Result"(TRUE ("St1 Test Result")) -> ()
                    }
                    frame "101" {
                      "St2 Test Result" <- FALSE ("St1 Test Result")
                    }
                  }
                  n115 = case shown="\"100\", Default" w183 {
                    frame "100", Default {
                      n116 = local write "St3 Status"(FALSE ("Running?")) -> ()
                    }
                    frame "010" {
                      "St3 Status" <- TRUE ("Running?")
                    }
                    frame "110" {
                      n117 = local write "St3 Test Result"(TRUE ("St1 Test Result")) -> ()
                    }
                    frame "101" {
                      "St3 Test Result" <- FALSE ("St1 Test Result")
                    }
                  }
                }
              }
            }
          }
        }
      }
      event "Robot Available": Value Change {
        n118 = event-data() -> ()  [unwired: 1 in, 6 out]
        n119 = Boolean To (0,1)(Boolean="Robot Available") -> (0, 1=w221:i16)
        n120 = local write "Robot_Available"(w221) -> ()
      }
      event "Start Test": Value Change {
        n121 = event-data() -> ("NewVal"=w223:bool)  [unwired: 1 in, 5 out]
        n122 = Boolean To (0,1)(Boolean=w223) -> (0, 1=w224:i16)
        n123 = local write "Start_Test"(w224) -> ()
      }
      event "Scan Trigger": Value Change {
        n124 = event-data() -> ("NewVal"=w225:bool)  [unwired: 1 in]
        n125 = Boolean To (0,1)(Boolean=w225) -> (0, 1=w226:i16)
        n126 = local write "Scan_Trigger"(w226) -> ()
      }
      event "Station No Start Stop Test": Value Change {
        n127 = event-data() -> ("NewVal"=w227:T3)  [unwired: 1 in]
        n128 = local write "Station_No_Start_Stop_Test"(w227) -> ()
      }
      event "PC ACK Read Tags": Value Change {
        n129 = event-data() -> ()  [unwired: 1 in, 6 out]
        n130 = local write "PC_ACK_Read_Tags"("PC ACK Read Tags") -> ()
      }
      event "Task_Available_for_Robot", "New_Serial", "Serial_Adapter_Size", "Station_Number", "Rerun", "Invalid_SNo", "PC_ACK_Read_Tags", "Serial_Displacement_Size", "Serial_Flange_Size", "Test_Result": Value Change {
        n131 = event-data() -> ()  [unwired: 1 in, 6 out]
        n132 = To Unsigned Long Integer(number="Station_Number") -> (unsigned 32bit integer=w236:u32)
        n133 = To Unsigned Long Integer(number="Task_Available_for_Robot") -> (unsigned 32bit integer=w248:u32)
        n134 = To Unsigned Long Integer(number="New_Serial") -> (unsigned 32bit integer=w247:u32)
        n135 = To Unsigned Long Integer(number="Test_Result") -> (unsigned 32bit integer=w241:u32)
        n136 = To Unsigned Long Integer(number="Invalid_SNo") -> (unsigned 32bit integer=w232:u32)
        n137 = local write "PC ACK Read Tags"("PC_ACK_Read_Tags") -> ()
        n138 = To Unsigned Long Integer(number="Rerun") -> (unsigned 32bit integer=w235:u32)
        n139 = Number To Decimal String(number=w236) -> (decimal integer string=→"Station Number":string)  [unwired: 1 in]
        n140 = Not Equal To 0?(x=w248) -> (x != 0?=→"Task Available for Robot?":bool)
        n141 = Not Equal To 0?(x=w247) -> (x != 0?=→"New Serial Task?":bool)
        n142 = Not Equal To 0?(x=w241) -> (x != 0?=→"Test Result":bool)
        n143 = Not Equal To 0?(x=w232) -> (x != 0?=→"Invalid Serial Number":bool)
        n144 = Not Equal To 0?(x=w235) -> (x != 0?=→"Rerun?":bool)
        "Serial Adapter Plate Size" <- "Serial_Adapter_Size"
        "Serial Displacement Size" <- "Serial_Displacement_Size"
        "Serial Flange Size" <- "Serial_Flange_Size"
      }
      event "Stop Test": Value Change {
        n145 = event-data() -> ("NewVal"=w251:bool)  [unwired: 1 in, 5 out]
        n146 = Boolean To (0,1)(Boolean=w251) -> (0, 1=w252:i16)
        n147 = local write "Stop_Test"(w252) -> ()
      }
      event "Trigger Robot Controller State": Value Change {
        n148 = event-data() -> ()  [unwired: 1 in, 6 out]
        n149 = call "ALTS Robot Cotroller Queue Reference.vi"() -> ("error out"=w255:errorcluster, "queue out"=w254:refnum<queue>)  [unwired: 10 in]
        n150 = Flush Queue(queue=w254, error in (no error)=w255) -> (error out=w253:errorcluster)  [unwired: 2 out]
        n151 = call "ALTS Robot controller Enqueue element.vi"("error in"=w253, "element"="Enum") -> ()  [unwired: 9 in, 1 out]
      }
      event "stop": Value Change {
        n152 = event-data() -> ()  [unwired: 1 in, 6 out]
      }
      event Timeout {
        n153 = event-data() -> ()  [unwired: 1 in, 3 out]
      }
    }
  }
  n154 = while {
    tunnel: "error in" -> [w266]
    tunnel: [w265] -> w19
    shift-right: [w269] -> _
    shift-left: "" -> [w267]
    tunnel: w2 -> [w264]
    stop <- "stop" stop-if-true
    n155 = event shown="[0] Timeout" {
      selector: _ -> [_ _ _ _]
      dyn-events: _ -> [_ _ _ _]
      timeout: 100 -> [_ _ _ _]
      tunnel: [w272 w314 w331 w349] -> w269
      tunnel: w267 -> [w273 w313 w330 w350]
      tunnel: w266 -> [w278 _ _ _]
      tunnel: [w277 _ _ _] -> w265
      tunnel: w264 -> [w274 _ _ _]
      event Timeout {
        n156 = event-data() -> ()  [unwired: 1 in, 1 out]
        n157 = for {
          tunnel: w274 -> [w312] mode=indexing
          tunnel: [w311] -> w275 mode=indexing
          n158 = property class="Ctl"(reference=w312) -> ("Value"=w311:variant)  [unwired: 1 in, 2 out]
        }
        n159 = call "SLL DE DI LV2 Global.vi"("DI State Array"="DI Array", "Option"=SLL_DE_DI_Global_Options."Write Array", "error in (no error)"=w278, "DI Channel Name Array"="DI Channel Name Array") -> ("error out"=w283:errorcluster)  [unwired: 4 in, 3 out]
        n160 = call "SLL DE DO LV2 Global.vi"("DO Option"=SLL_DE_DO_Global_Options."Read Full Status", "Error In"=w283) -> ("error out"=w277:errorcluster, "Digital Array Status"=w284:bool[])  [unwired: 6 in, 2 out]
        n161 = feedback-in #1(w275) -> ()
        n162 = feedback #1() -> (w276:variant[])  [unwired: 1 in]
        n163 = Not Equal?(x=w276, y=w275) -> (x != y?=w271:bool[])
        n164 = for {
          tunnel: w274 -> [w292]
          shift-right: [w287] -> _
          shift-left: w271 -> [w288]
          tunnel: w271 -> [_] mode=indexing
          shift-right: [w290] -> w272
          shift-left: w273 -> [w291]
          n165 = Search 1D Array(1D array=w288, element=TRUE) -> (index of element=w286:i32)  [unwired: 1 in]
          n166 = Index Array(array=w292, index=w286) -> (element=w289:refnum<vi>)
          n167 = case shown="-1, Default" w286 {
            tunnel: [w294 w302] -> w290
            tunnel: w291 -> [w294 w301]
            tunnel: w289 -> [_ w298]
            frame -1, Default {
            }
            frame 0.. {
              n168 = property class="Ctl"(reference=w298) -> ("Value"=w300:variant, "ClassName"=w297:string, "Label.Text"=w295:string)  [unwired: 1 in, 2 out]
              n169 = case shown="Default" w297 {
                tunnel: w300 -> [w305 w309]
                tunnel: [w304 w307] -> w299
                frame "String" {
                  n170 = Variant To Data(type="" ("concatenated string"), Variant=w305) -> (data=w304:string)  [unwired: 1 in, 1 out]
                }
                frame Default {
                  n171 = Variant To Data(type=0 ("concatenated string"), Variant=w309) -> (data=w308:i32)  [unwired: 1 in, 1 out]
                  n172 = Number To Decimal String(number=w308) -> (decimal integer string=w307:string)  [unwired: 1 in]
                }
              }
              n173 = Concatenate Strings(w301, w295, " = " ("string"), w299, "\n") -> (w302:string)
            }
          }
          n174 = Replace Array Subset(array=w288, new element=FALSE ("new element/subarray"), index=w286) -> (w287:bool[])
        }
        n175 = property on="DO Status" class="Arr (strict)"("Val(Sgnl)"=w284) -> ()  [unwired: 2 in, 2 out]
      }
      event "DI Array": Value Change {
        n176 = event-data() -> ("OldVal"=w322:bool[], "NewVal"=w321:bool[])  [unwired: 1 in, 4 out]
        n177 = Not Equal?(x=w322, y=w321) -> (x != y?=w320:bool[])
        n178 = property on="DI Channel Name" class="Enum (strict)"() -> ("Strings []"=w318:string[])  [unwired: 2 in, 2 out]
        n179 = Search 1D Array(1D array=w320, element=TRUE) -> (index of element=w317:i32)  [unwired: 1 in]
        n180 = Index Array(array=w318, index=w317) -> (element=w315:string)
        n181 = Concatenate Strings(w313, w315, "\n") -> (w314:string)
      }
      event "DO Status": Value Change {
        n182 = event-data() -> ("OldVal"=w334:bool[], "NewVal"=w328:bool[])  [unwired: 1 in]
        n183 = Not Equal?(x=w334, y=w328) -> (x != y?=w333:bool[])
        n184 = property on="DO Channel Name" class="Enum (strict)"() -> ("Strings []"=w329:string[])  [unwired: 2 in, 2 out]
        n185 = Search 1D Array(1D array=w333, element=TRUE) -> (index of element=w327:i32)  [unwired: 1 in]
        n186 = Index Array(array=w328, index=w327) -> (element=w326:bool)
        n187 = Select(t="TRUE", s=w326, f="FALSE") -> (s? t:f=w323:string)
        n188 = case shown="0.." w327 {
          tunnel: w327 -> [_ w343]
          tunnel: [w335 w340] -> w331
          tunnel: w329 -> [_ w339]
          tunnel: w330 -> [w335 w338]
          tunnel: w323 -> [_ w336]
          frame -1, Default {
          }
          frame 0.. {
            n189 = Index Array(array=w339, index=w343) -> (element=w341:string)
            n190 = Concatenate Strings(w338, w341, " = " ("string"), w336, "\n") -> (w340:string)
          }
        }
      }
      event "Robot_Available", "Start_Test", "Stop_Test", "Scan_Trigger", "Station_No_Start_Stop_Test": Value Change {
        n191 = event-data() -> ("CtlRef"=w351:refnum<vi>)  [unwired: 1 in, 5 out]
        n192 = property class="DigNum (strict)"(reference=w351) -> ("Label.Text"=w348:string, "Value"=w347:dbl)  [unwired: 1 in, 2 out]
        n193 = Number To Decimal String(number=w347) -> (decimal integer string=w346:string)  [unwired: 1 in]
        n194 = Concatenate Strings(w350, w348, " = " ("string"), w346, "\n") -> (w349:string)
      }
    }
    "String" <- w269
    n195 = call "ALTS-2015 LV2GBL Station Info.vi"("Options"=ALTS-2015_LV2GBL_Station_Info_Options."Read", "Station Cluster"="Station_No_Start_Stop_Test") -> ("error out"=w260:errorcluster, "Station Details"=w263:T10)  [unwired: 7 in, 1 out]
    n196 = Unbundle By Name(w263) -> ("Station Number"=→"Station Number":string, "Test Type"=→"Test Type":i32)
    n197 = call <vilib>:"Clear Errors.vi"("error in (no error)"=w260) -> ()  [unwired: 6 in, 1 out]
  }
  "error out" <- w19
  n198 = for {
    N: 24 -> [_]
    tunnel: [w352] -> w17 mode=indexing
    i -> [w352]
  }
  n199 = for {
    N: 28 -> [_]
    tunnel: [w353] -> w14 mode=indexing
    i -> [w353]
  }
  n200 = property on="DO Channel Name Array" class="Arr (strict)"("Value"=w17) -> ()  [unwired: 2 in, 2 out]
  n201 = property on="DI Channel Name Array" class="Arr (strict)"("Value"=w14) -> ()  [unwired: 2 in, 2 out]
  n202 = control-ref of="This VI"() -> (w13:refnum<vi>)
  n203 = invoke class="VI" method="Default Vals.Reinit All"(reference=w13) -> ()  [unwired: 2 in, 3 out]
